vi "Read Processed Request.vi"(0 "Version Ref":refnum<vi>, 5 "Produced Methods":u16(ring) items=["box", "EtFlocSedFi", "EtFlocSedFiLow", "Flocculator", "lfom", "Sedimentation Tank", "SedTank", "SRSF"], 11 "error in (no error)":errorcluster, 12 "Request Number":i32) -> (1 "RequestID":string, 3 "formdata":T3, 6 "User and project info":T2, 8 "Mathcad Results":T2, 10 "timing":T1, 13 "time stamp":timestamp, 14 "Number of designs":i32, 15 "error out":errorcluster)   [LabVIEW 2011]
uses:
  user project design.ctl
  Variable cluster.ctl
  Design Server.lvlib
panel:
  out "appended path":path
  out "sorted array":cluster{"last mod":timestamp, string}[](array[cluster])
  in  "NewYear2012":timestamp=timestamp(3408238800 s since 1904-01-01)
  in  "request datatype":T3
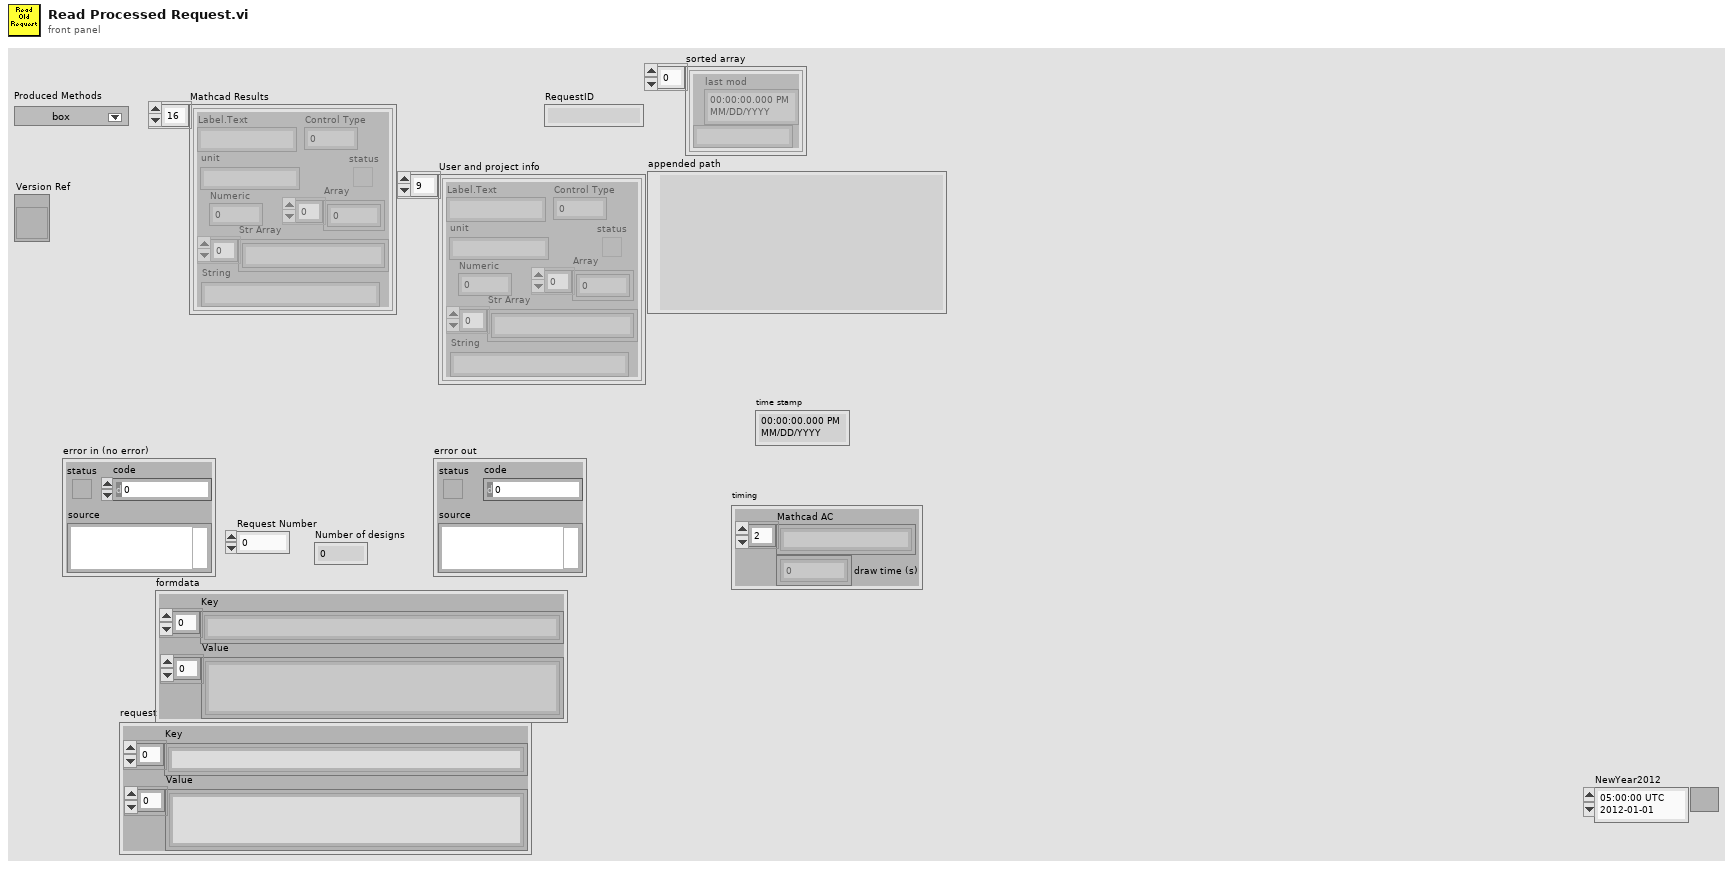
[diagram p1: front panel]
types:
  T1 = cluster{"draw time (s)":dbl[], "Mathcad AC":string[]}
  T2 = typedef "Design Server.lvlib/Variable cluster.ctl" = cluster{"Label.Text":string, "Control Type":u32, "Numeric":dbl, "Array":dbl[], "status":bool, "Str Array":string[], "String":string, "unit":string}[]
  T3 = typedef "Design Server.lvlib/user project design.ctl" = cluster{"Key":string[], "Value":string[]}
  T4 = enum16{"open", "replace", "create", "open or create", "replace or create", "replace or create with confirmation"}
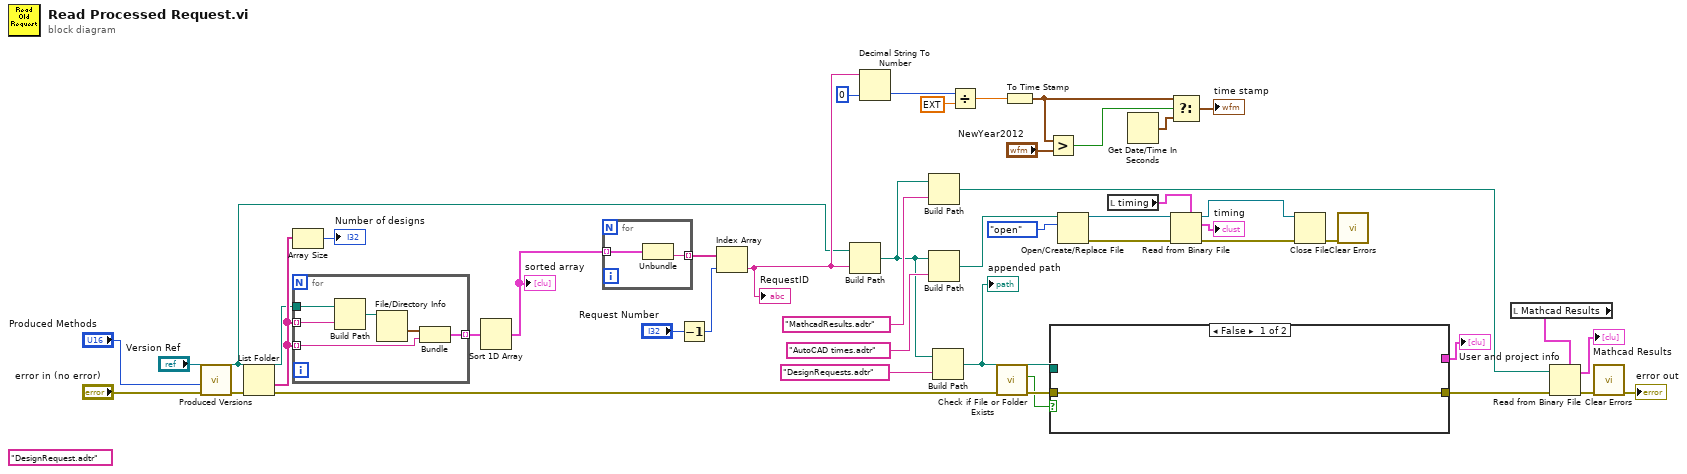
[diagram p0: block diagram]
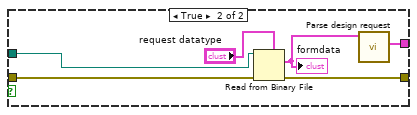
[diagram p2: hidden frame]
diagram:
  (unwired) "DesignRequest.adtr"
  n1 = call "Produced Versions.vi"("error in"="error in (no error)", "Produced Method"="Produced Methods", "Version Ref"="Version Ref") -> ("error out"=w2:errorcluster, "Designs in Method version"=w4:path)  [unwired: 7 in]
  n2 = List Folder(path=w4, error in=w2) -> (path out=w11:path, folder names=w12:string[], error out=w10:errorcluster)  [unwired: 2 in, 1 out]
  n3 = Array Size(array=w12) -> (size(s)=→"Number of designs":i32)
  n4 = for {
    tunnel: w11 -> [w51]
    tunnel: w12 -> [w52] mode=indexing
    tunnel: [w54] -> w17 mode=indexing
    tunnel: w12 -> [w49] mode=indexing
    n5 = Build Path(base path=w51, name or relative path=w49) -> (appended path=w50:path)
    n6 = File/Directory Info(path=w50) -> (last mod=w53:timestamp)  [unwired: 1 in, 6 out]
    n7 = Bundle("last mod"=w53, w52) -> (w54:cluster{"last mod":timestamp, string})  [unwired: 1 in]
  }
  n8 = Sort 1D Array(array=w17) -> (sorted array=w16:cluster{"last mod":timestamp, string}[])
  "sorted array" <- w16
  n9 = for {
    tunnel: w16 -> [w56] mode=indexing
    tunnel: [w55] -> w15 mode=indexing
    n10 = Unbundle(w56) -> (w55:string)  [unwired: 1 out]
  }
  n11 = Decrement(x="Request Number") -> (x-1=w13:i32)
  n12 = Index Array(array=w15, index=w13) -> (element=w19:string)
  "RequestID" <- w19
  n13 = Build Path(base path=w4, name or relative path=w19) -> (appended path=w31:path)
  n14 = Decimal String To Number(string=w19, default (0L)=i64 0 ("default (0 I32)")) -> (number=w25:i64)  [unwired: 1 in, 1 out]
  n15 = Build Path(base path=w31, name or relative path="MathcadResults.adtr") -> (appended path=w44:path)
  n16 = Build Path(base path=w31, name or relative path="AutoCAD times.adtr") -> (appended path=w36:path)
  n17 = Build Path(base path=w31, name or relative path="DesignRequests.adtr") -> (appended path=w8:path)
  "appended path" <- w8
  n18 = Divide(x=w25, y=ext 100.0) -> (x/y=w26:ext)
  n19 = call <vilib>:"Check if File or Folder Exists.vi"("error in (no error)"=w10, "path"=w8) -> ("error out"=w9:errorcluster, "file or folder exists?"=w1:bool, "dup path"=w7:path)  [unwired: 7 in]
  n20 = To Time Stamp(1:w26) -> (0:w21:timestamp)
  n21 = Greater?(x=w21, y="NewYear2012") -> (0:w22:bool)
  n22 = case shown="False" w1 {
    tunnel: [_ w63] -> w48
    tunnel: [w57 w61] -> w41
    tunnel: w9 -> [w57 w59]
    tunnel: w7 -> [_ w58]
    frame False {
    }
    frame True {
      n23 = Read from Binary File(5:"request datatype", 8:w59, 11:w58) -> (0:w61:errorcluster, 2:w60:T3)  [unwired: 3 in, 2 out]
      "formdata" <- w60
      n24 = call "Parse design request.vi"("Request"=w60) -> ("User and project info"=w63:T2)  [unwired: 7 in, 3 out]
    }
  }
  "User and project info" <- w48
  n25 = Open/Create/Replace File(file path (use dialog)=w36, operation (0:open)=T4."open") -> (refnum out=w34:refnum<file>, error out=w38:errorcluster)  [unwired: 4 in, 1 out]
  n26 = local read "timing"() -> (w28:T1)
  n27 = Get Date/Time In Seconds() -> (seconds since 1Jan1904=w20:timestamp)
  n28 = Select(t=w21, s=w22, f=w20) -> (s? t:f=→"time stamp":timestamp)
  n29 = Read from Binary File(5:w28, 8:w38, 11:w34) -> (0:w33:errorcluster, 2:→"timing":T1, 3:w32:refnum<file>)  [unwired: 3 in, 1 out]
  n30 = Close File(refnum=w32, error in=w33) -> (error out=w30:errorcluster)  [unwired: 1 out]
  n31 = call <vilib>:"Clear Errors.vi"("error in (no error)"=w30) -> ()  [unwired: 6 in, 1 out]
  n32 = local read "Mathcad Results"() -> (w43:T2)
  n33 = Read from Binary File(5:w43, 8:w41, 11:w44) -> (0:w40:errorcluster, 2:→"Mathcad Results":T2)  [unwired: 3 in, 2 out]
  n34 = call <vilib>:"Clear Errors.vi"("error in (no error)"=w40) -> ("error out"=→"error out":errorcluster)  [unwired: 6 in]
